vi "ReadTriggerOutputNode.vi"(8 "Error In":errorcluster, 11 "Keithley2602 Node In":refnum<k20>) -> (0 "Error Out":errorcluster, 2 "Output Trigger Configuration":T1={"Type"=enum."None", "Delay (ms)"=0, "Digital IO Line (1-14)"=2, "Digital IO Mode"=enum."Falling", "Digital IO Pulse Width (sec)"=0.0} {"Digital IO Line (1-14)" min=1 max=14 step=1}, 3 "Keithley2602 Node Out":refnum<k20>)   [LabVIEW 2013]
uses:
  TriggerOutputConfiguration.ctl
  TriggerOutputType.ctl
  driver/Public/Controls/TriggerMode.ctl
  driver/Keithley-2602.lvlib
  <vilib>/xml/NI_XML.lvlib
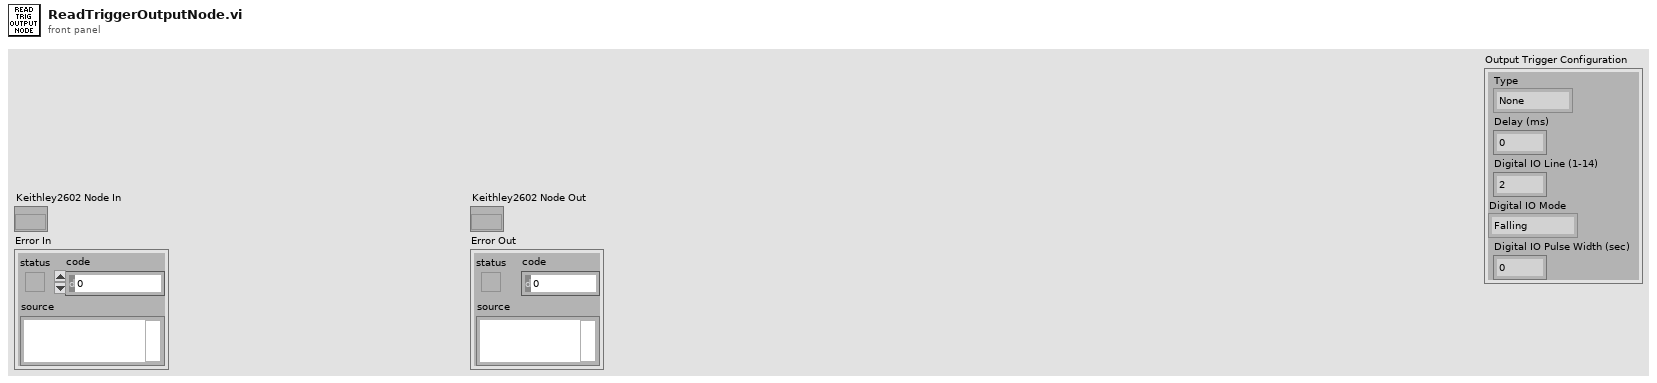
[diagram p1: front panel]
types:
  T1 = typedef "TriggerOutputConfiguration.ctl" = cluster{"Type":T2, "Delay (ms)":u32, "Digital IO Line (1-14)":u8, "Digital IO Mode":T3, "Digital IO Pulse Width (sec)":dbl}
  T2 = typedef "TriggerOutputType.ctl" = enum16{"None", "Digital IO", "Bus"}
  T3 = typedef "Keithley-2602.lvlib/TriggerMode.ctl" = enum16{"Falling", "Rising", "Either", "Synchronous"}
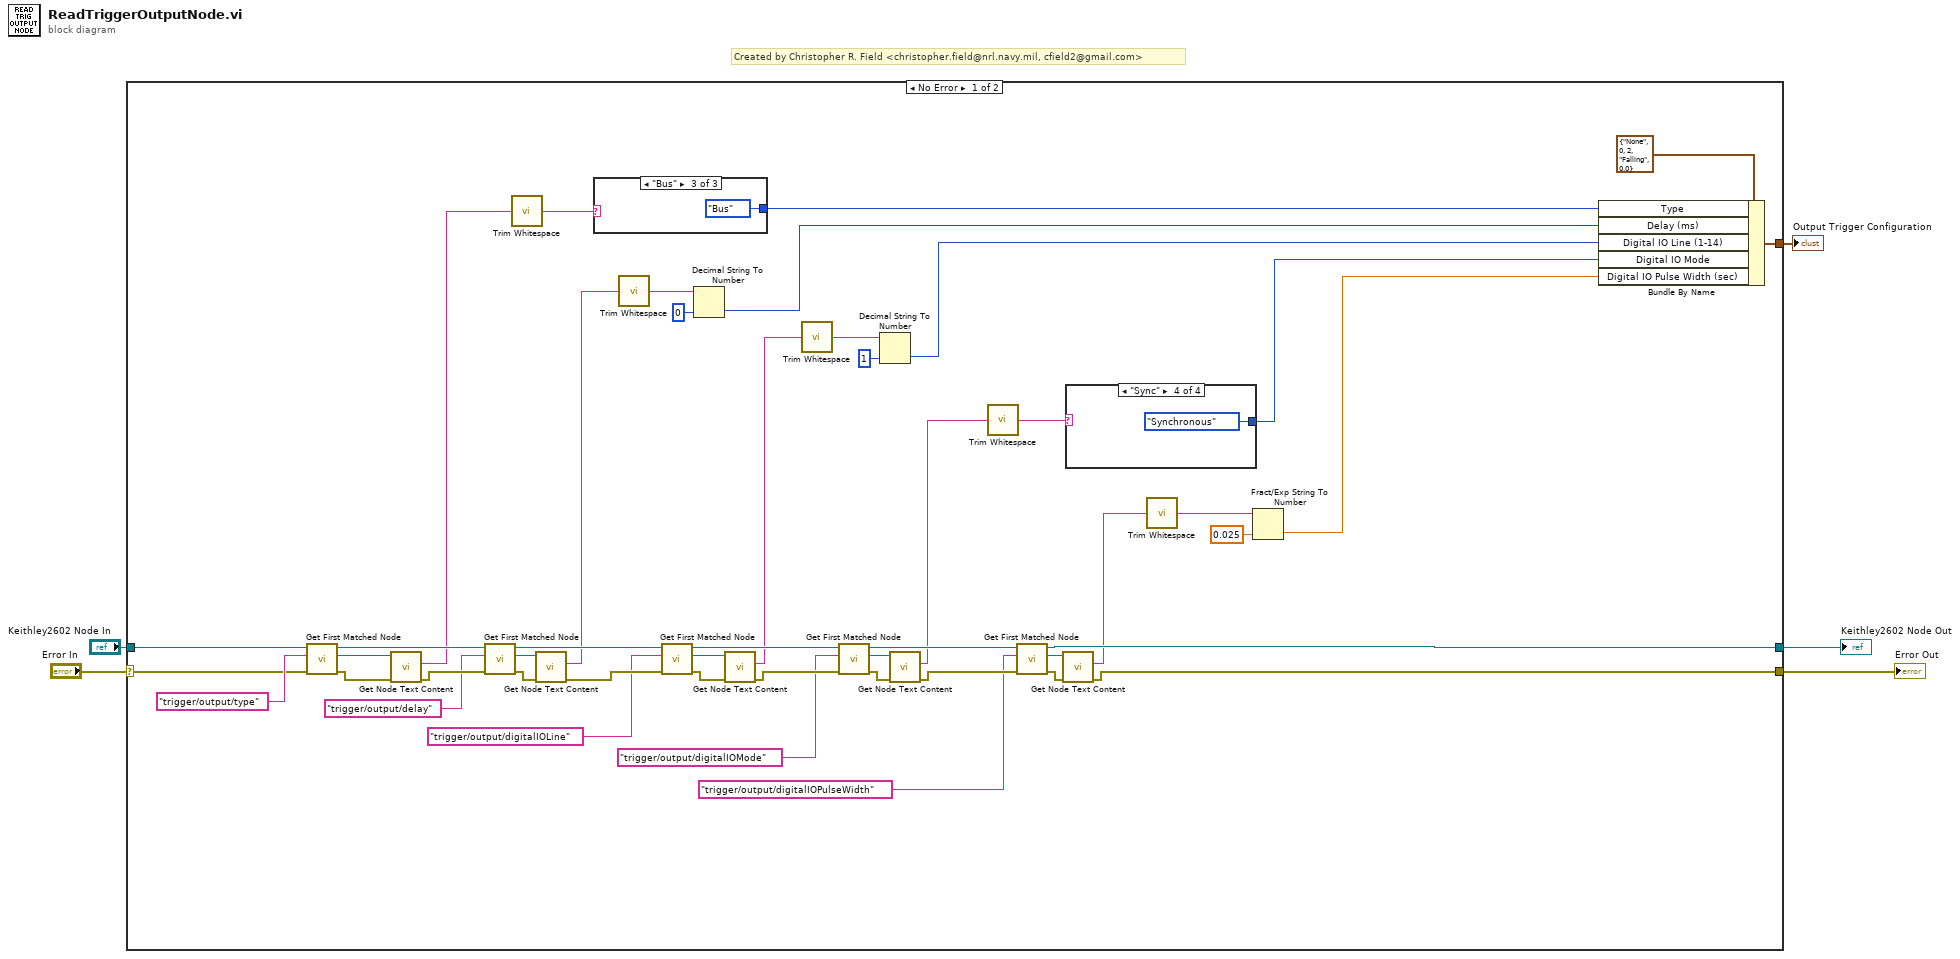
[diagram p0: block diagram]
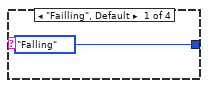
[diagram p2: hidden frame]
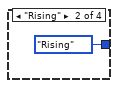
[diagram p3: hidden frame]
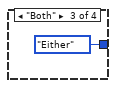
[diagram p4: hidden frame]
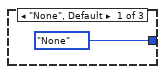
[diagram p5: hidden frame]
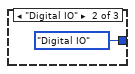
[diagram p6: hidden frame]
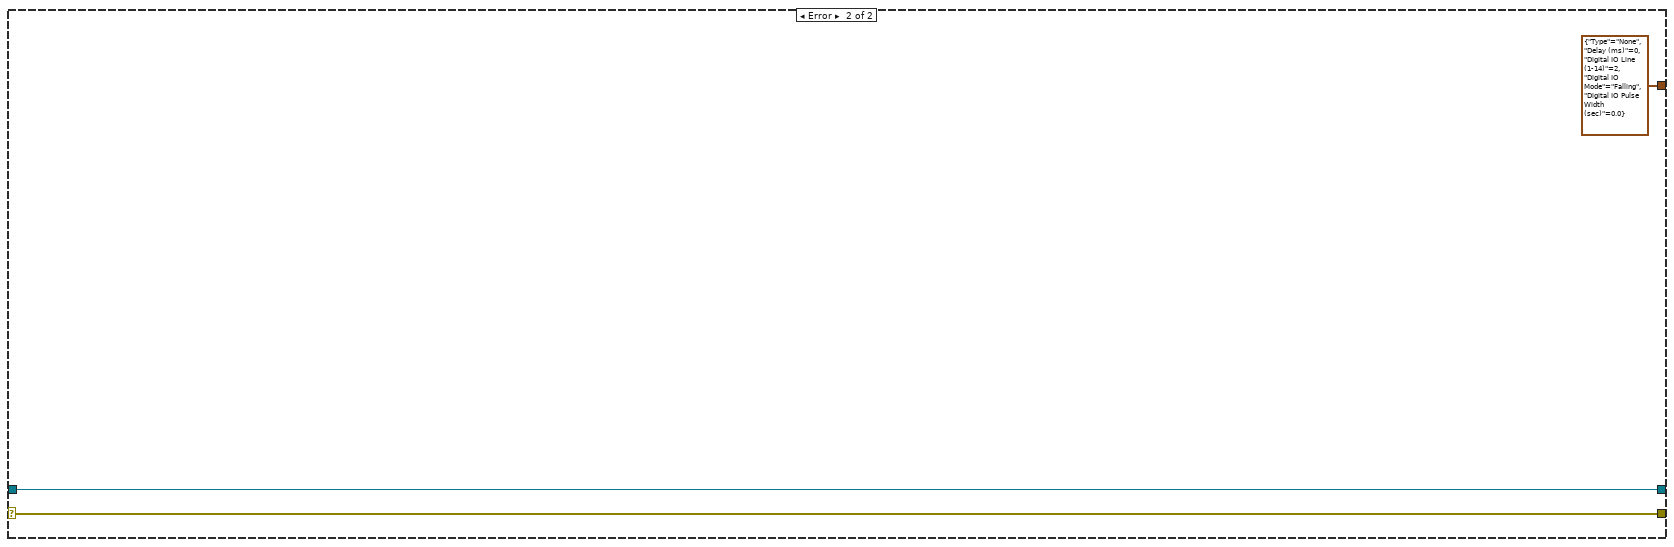
[diagram p7: hidden frame]
diagram:
  # "Created by Christopher R. Field <christopher.field@nrl.navy.mil, cfield2@gmail.com>"
  n1 = case shown="No Error" "Error In" {
    selector: "Error In" -> [w24 w61]
    tunnel: "Keithley2602 Node In" -> [w25 w62]
    tunnel: [w22 w62] -> w3
    tunnel: [w23 w61] -> w2
    tunnel: [w51 T1 {"Type"=enum."None", "Delay (ms)"=0, "Digital IO Line (1-14)"=2, "Digital IO Mode"=enum."Falling", "Digital IO Pulse Width (sec)"=0.0} ("Output Trigger Configuration")] -> w1
    frame No Error {
      n2 = call <vilib>:"Get First Matched Node.vi"("error in (no error)"=w24, "XPath expression"="trigger/output/type", "node in"=w25) -> ("error out"=w48:errorcluster, "node result"=w49:refnum<k20>, "node out"=w47:refnum<k20>)  [unwired: 6 in]
      n3 = call <vilib>:"Get Node Text Content.vi"("error in (no error)"=w48, "node in"=w49) -> ("error out"=w46:errorcluster, "node text"=w14:string)  [unwired: 7 in, 1 out]
      n4 = call <vilib>:"Get First Matched Node.vi"("error in (no error)"=w46, "XPath expression"="trigger/output/delay", "node in"=w47) -> ("error out"=w44:errorcluster, "node result"=w45:refnum<k20>, "node out"=w41:refnum<k20>)  [unwired: 6 in]
      n5 = call <vilib>:"Trim Whitespace.vi"("string"=w14) -> ("trimmed string"=w15:string)  [unwired: 1 in]
      n6 = call <vilib>:"Get Node Text Content.vi"("error in (no error)"=w44, "node in"=w45) -> ("error out"=w40:errorcluster, "node text"=w12:string)  [unwired: 7 in, 1 out]
      n7 = case shown="\"Bus\"" w15 {
        tunnel: [TriggerOutputType."None" ("Type") TriggerOutputType."Digital IO" ("Type") TriggerOutputType."Bus" ("Type")] -> w17
        frame "None", Default {
        }
        frame "Digital IO" {
        }
        frame "Bus" {
        }
      }
      n8 = call <vilib>:"Trim Whitespace.vi"("string"=w12) -> ("trimmed string"=w13:string)  [unwired: 1 in]
      n9 = call <vilib>:"Get First Matched Node.vi"("error in (no error)"=w40, "XPath expression"="trigger/output/digitalIOLine", "node in"=w41) -> ("error out"=w38:errorcluster, "node result"=w39:refnum<k20>, "node out"=w35:refnum<k20>)  [unwired: 6 in]
      n10 = Decimal String To Number(string=w13, default (0L)=u32 0 ("default (0 I32)")) -> (number=w18:u32)  [unwired: 1 in, 1 out]
      n11 = call <vilib>:"Get Node Text Content.vi"("error in (no error)"=w38, "node in"=w39) -> ("error out"=w34:errorcluster, "node text"=w10:string)  [unwired: 7 in, 1 out]
      n12 = call <vilib>:"Trim Whitespace.vi"("string"=w10) -> ("trimmed string"=w11:string)  [unwired: 1 in]
      n13 = call <vilib>:"Get First Matched Node.vi"("error in (no error)"=w34, "XPath expression"="trigger/output/digitalIOMode", "node in"=w35) -> ("error out"=w31:errorcluster, "node result"=w32:refnum<k20>, "node out"=w30:refnum<k20>)  [unwired: 6 in]
      n14 = Decimal String To Number(string=w11, default (0L)=u32 1 ("default (0 I32)")) -> (number=w19:u32)  [unwired: 1 in, 1 out]
      n15 = call <vilib>:"Get Node Text Content.vi"("error in (no error)"=w31, "node in"=w32) -> ("error out"=w29:errorcluster, "node text"=w9:string)  [unwired: 7 in, 1 out]
      n16 = call <vilib>:"Trim Whitespace.vi"("string"=w9) -> ("trimmed string"=w8:string)  [unwired: 1 in]
      n17 = call <vilib>:"Get First Matched Node.vi"("error in (no error)"=w29, "XPath expression"="trigger/output/digitalIOPulseWidth", "node in"=w30) -> ("error out"=w26:errorcluster, "node result"=w27:refnum<k20>, "node out"=w22:refnum<k20>)  [unwired: 6 in]
      n18 = call <vilib>:"Get Node Text Content.vi"("error in (no error)"=w26, "node in"=w27) -> ("error out"=w23:errorcluster, "node text"=w6:string)  [unwired: 7 in, 1 out]
      n19 = case shown="\"Sync\"" w8 {
        tunnel: [TriggerMode."Falling" ("Digital IO Mode") TriggerMode."Rising" ("Digital IO Mode") TriggerMode."Either" ("Digital IO Mode") TriggerMode."Synchronous" ("Digital IO Mode")] -> w21
        frame "Failling", Default {
        }
        frame "Rising" {
        }
        frame "Both" {
        }
        frame "Sync" {
        }
      }
      n20 = call <vilib>:"Trim Whitespace.vi"("string"=w6) -> ("trimmed string"=w7:string)  [unwired: 1 in]
      n21 = Fract/Exp String To Number(string=w7, default (0 dbl)=0.025 ("default (0 DBL)")) -> (number=w20:dbl)  [unwired: 2 in, 1 out]
      n22 = Bundle By Name(cluster=T1 {"Type"=enum."None", "Delay (ms)"=0, "Digital IO Line (1-14)"=2, "Digital IO Mode"=enum."Falling", "Digital IO Pulse Width (sec)"=0.0} ("Output Trigger Configuration"), "Type"=w17, "Delay (ms)"=w18, "Digital IO Line (1-14)"=w19, "Digital IO Mode"=w21, "Digital IO Pulse Width (sec)"=w20) -> (w51:T1)
    }
    frame Error {
    }
  }
  "Keithley2602 Node Out" <- w3
  "Error Out" <- w2
  "Output Trigger Configuration" <- w1
